vi "Read Value from Property Key.vi"(8 "error in (no error)":errorcluster, 10 "Key":string, 11 "Service in":refnum<class "Service.lvclass">) -> (0 "error out":errorcluster, 3 "Value":variant)   [LabVIEW 2024, in "Ramses Framework.lvlib" / "Service.lvclass"]
uses:
  Service.lvclass
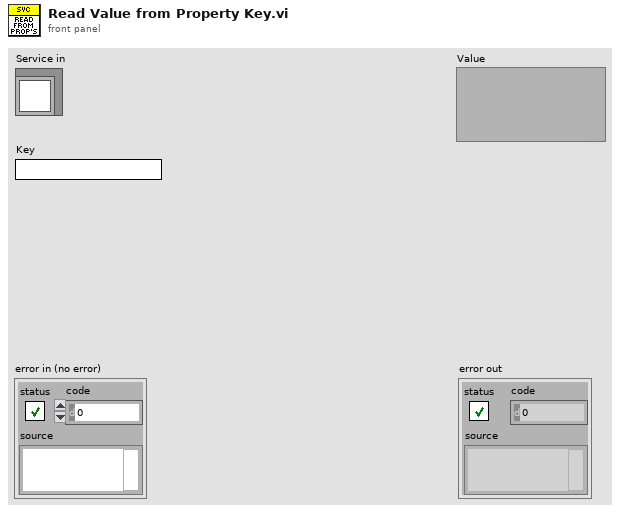
[diagram p1: front panel]
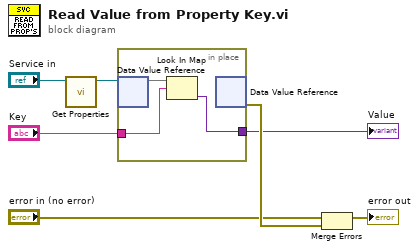
[diagram p0: block diagram]
diagram:
  n1 = call "Get Properties.vi"("Service in"="Service in") -> ("Properties"=w5:refnum<data-value>)  [unwired: 9 in, 1 out]
  n2 = in-place {
    in-place-border: [w8] -> w1
    in-place-border: "Key" -> [w9]
    n3 = in-place-dvr #1(w5) -> (w10:map{string, variant})  [unwired: 1 out]
    n4 = Look In Map(map=w10, key=w9) -> (value=w8:variant)  [unwired: 1 in, 1 out]
    n5 = in-place-dvr #1() -> (w3:errorcluster)  [unwired: 1 in, 1 out]
  }
  "Value" <- w1
  n6 = Merge Errors("error in (no error)", w3) -> (→"error out":errorcluster)
